vi "Print Document.vi"(8 "error in (no error)":errorcluster, 9 "number of copies (1)":i16=1, 10 "printer name (default)":string, 11 "Document in":refnum<class "Document.lvclass">) -> (0 "error out":errorcluster, 3 "Document out":refnum<class "Document.lvclass">)   [LabVIEW 2017, in "LabVIEW NPOI.lvlib" / "Document.lvclass"]
uses:
  Document.lvclass
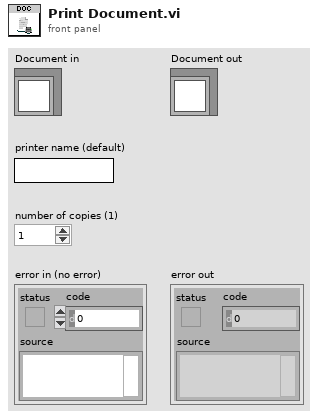
[diagram p1: front panel]
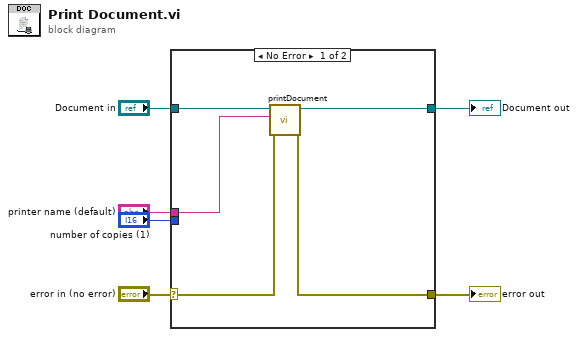
[diagram p0: block diagram]
diagram:
  n1 = case shown="No Error" "error in (no error)" {
    selector: "error in (no error)" -> [w9 w13]
    tunnel: [w8 w13] -> w5
    tunnel: [w10 w12] -> w3
    tunnel: "Document in" -> [w11 w12]
    tunnel: "printer name (default)" -> [w7 _]
    tunnel: "number of copies (1)" -> [_ _]
    frame No Error {
      n2 = call-dynamic "printDocument.vi"("error in (no error)"=w9, "printer name (default)"=w7, "Document in"=w11) -> ("error out"=w8:errorcluster, "Document out"=w10:refnum<class "Document.lvclass">)  [unwired: 7 in]
    }
    frame Error {
    }
  }
  "error out" <- w5
  "Document out" <- w3
